vi "Initialize.vi"(7 "Baud Rate (3: 57600)":i32(ring)=3 items=["300", "1200", "9600", "57600 (USB Only)"], 8 "error in (no error)":errorcluster, 9 "Reset (True)":bool=TRUE, 10 "ID Query (True)":bool=TRUE, 11 "VISA resource name":refnum<visa-resource-name>) -> (0 "error out":errorcluster, 3 "VISA resource name out":refnum<visa-resource-name>)   [LabVIEW 2015, in "Lake Shore 372.lvlib"]
doc: "Establishes communication with the instrument and optionally performs an instrument identification query and/or an instrument reset. It also places the instrument in a default state needed for other instrument driver operations. Therefore, call this VI before calling other instrument driver VIs for this instrument. Generally, you need to call the Initialize VI only once at the beginning of an application.\n\nNOTE: If you do not want the instrument to reset to its default setup state, you MUST set the Reset Defaults control to FALSE."
uses:
  <instrlib>/Lake Shore 372/Lake Shore 372.lvlib
panel:
  # "(c) 2015 Advint LLC. ALL RIGHTS RESERVED."
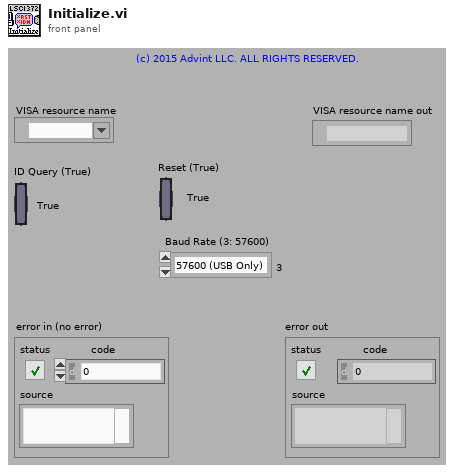
[diagram p1: front panel]
types:
  T1 = cluster{"Status":bool, "Code":i32, "Source (VI Name)":string}
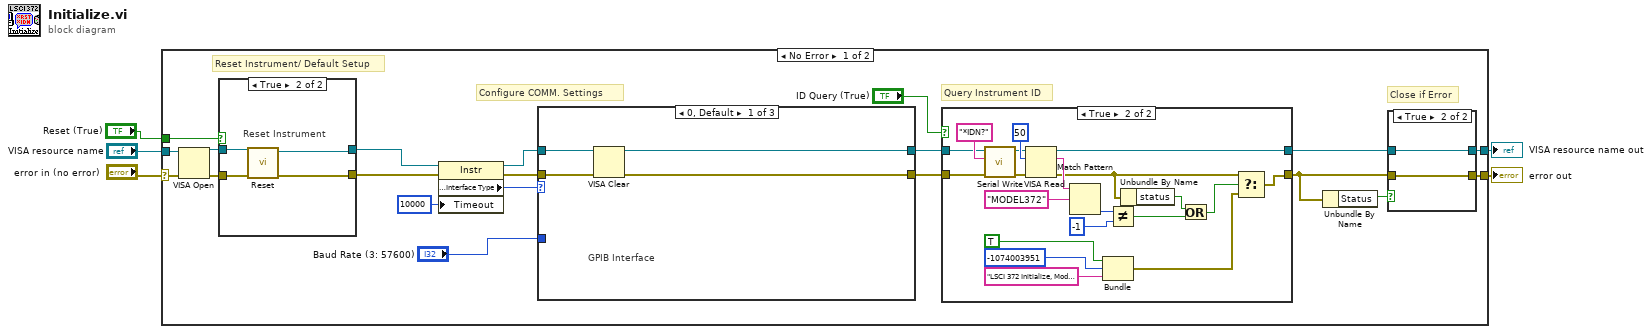
[diagram p0: block diagram]
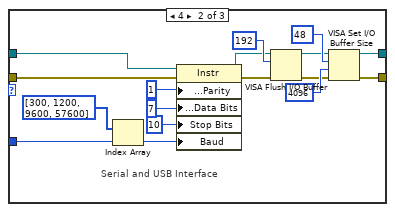
[diagram p2: hidden frame]
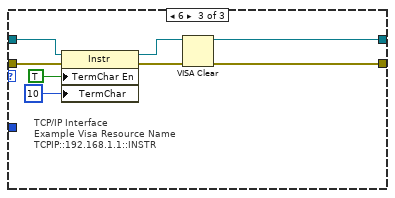
[diagram p3: hidden frame]
diagram:
  n1 = case shown="No Error" "error in (no error)" {
    selector: "error in (no error)" -> [w6 w87]
    tunnel: [w23 w88] -> w5
    tunnel: [w22 w87] -> w4
    tunnel: "Reset (True)" -> [w12 _]
    tunnel: "VISA resource name" -> [w7 w88]
    frame No Error {
      # "Configure COMM. Settings"
      # "Close if Error"
      # "Reset Instrument/ Default Setup"
      # "Query Instrument ID"
      n2 = VISA Open(error in (no error)=w6, VISA resource name=w7) -> (VISA resource name=w13:refnum<visa-resource-name>, error out=w14:errorcluster)  [unwired: 3 in]
      n3 = case shown="True" w12 {
        tunnel: w14 -> [w59 w63]
        tunnel: [w59 w61] -> w10
        tunnel: w13 -> [w60 w64]
        tunnel: [w60 w62] -> w11
        frame False {
          # "Do Not Reset \n  Instrument"
        }
        frame True {
          # "Reset Instrument"
          n4 = call <instrlib>:"Reset.vi"("error in (no error)"=w63, "VISA resource name"=w64) -> ("error out"=w61:errorcluster, "VISA resource name out"=w62:refnum<visa-resource-name>)  [unwired: 8 in]
        }
      }
      n5 = property on="Property Node" class="Instr"(reference=w11, error in=w10, "Timeout"=u32 10000 ("Tmo Value")) -> (reference out=w20:refnum<visa-resource-name>, error out=w21:errorcluster, "Interface Information:Interface Type"=w15:u16)
      n6 = case shown="0, Default" w15 {
        tunnel: w21 -> [w29 w43 w48]
        tunnel: [w27 w31 w51] -> w18
        tunnel: w20 -> [w28 w42 w49]
        tunnel: [w26 w30 w50] -> w19
        tunnel: "Baud Rate (3: 57600)" -> [_ w41 _]
        frame 0, Default {
          # "GPIB Interface"
          n7 = VISA Clear(VISA resource name=w28, error in (no error)=w29) -> (VISA resource name out=w26:refnum<visa-resource-name>, error out=w27:errorcluster)
        }
        frame 4 {
          # "Serial and USB Interface"
          n8 = Index Array(array=u32[] [300, 1200, 9600, 57600], index=w41) -> (element=w40:u32)
          n9 = property on="Property Node" class="Instr"(reference=w42, error in=w43, "Serial Settings:Parity"=1, "Serial Settings:Data Bits"=u16 7, "Stop Bits"=10, "Baud"=w40) -> (reference out=w32:refnum<visa-resource-name>, error out=w33:errorcluster)
          n10 = VISA Flush I/O Buffer(VISA resource name=w32, mask (16)=u16 192, error in (no error)=w33) -> (VISA resource name out=w36:refnum<visa-resource-name>, error out=w35:errorcluster)
          n11 = VISA Set I/O Buffer Size(VISA resource name=w36, mask (16)=u16 48, size (4096)=u32 4096 ("size (0)"), error in (no error)=w35) -> (VISA resource name out=w30:refnum<visa-resource-name>, error out=w31:errorcluster)
        }
        frame 6 {
          # "TCP/IP Interface\nExample Visa Resource Name\nTCPIP::192.168.1.1::INSTR"
          n12 = property on="Property Node" class="Instr"(reference=w49, error in=w48, "TermChar En"=TRUE, "TermChar"=u8 10 ("Message Based Settings:Termination Character")) -> (reference out=w52:refnum<visa-resource-name>, error out=w53:errorcluster)
          n13 = VISA Clear(VISA resource name=w52, error in (no error)=w53) -> (VISA resource name out=w50:refnum<visa-resource-name>, error out=w51:errorcluster)
        }
      }
      n14 = case shown="True" "ID Query (True)" {
        tunnel: [w65 w86] -> w9
        tunnel: [w66 w85] -> w8
        tunnel: w19 -> [w66 w71]
        tunnel: w18 -> [w65 w70]
        frame False {
        }
        frame True {
          n15 = call <instrlib>:"Serial Write.vi"("error in (no error)"=w70, "Write Buffer (\"\")"="*IDN?" ("ID Query"), "VISA resource name"=w71) -> ("error out"=w74:errorcluster, "VISA resource name out"=w73:refnum<visa-resource-name>)  [unwired: 6 in, 1 out]
          n16 = VISA Read(VISA resource name=w73, byte count=u32 50, error in (no error)=w74) -> (VISA resource name out=w85:refnum<visa-resource-name>, read buffer=w82:string, error out=w67:errorcluster)  [unwired: 1 out]
          n17 = Match Pattern(string=w82, regular expression="MODEL372") -> (offset past match=w69:i32)  [unwired: 1 in, 3 out]
          n18 = Bundle("Status"=TRUE, "Code"=-1074003951, "Source (VI Name)"="LSCI 372 Initialize, Model\nNumber not 372") -> (w77:T1)  [unwired: 1 in]
          n19 = Not Equal?(x=w69, y=-1) -> (x != y?=w83:bool)
          n20 = Unbundle By Name(w67) -> ("status"=w80:bool)
          n21 = Or(x=w80, y=w83) -> (x .or. y?=w81:bool)
          n22 = Select(t=w67, s=w81, f=w77) -> (s? t:f=w86:T1)
        }
      }
      n23 = Unbundle By Name(w9) -> ("Status"=w24:bool)
      n24 = case shown="True" w24 {
        tunnel: w8 -> [w56 w58]
        tunnel: w9 -> [w55 w57]
        tunnel: [w56 w58] -> w23
        tunnel: [w55 w57] -> w22
        frame False {
        }
        frame True {
        }
      }
    }
    frame Error {
    }
  }
  "VISA resource name out" <- w5
  "error out" <- w4
